vi "Get Settings File Name.vi"(7 "Source Path":path, 8 "error in (no error)":errorcluster) -> (0 "error out":errorcluster, 1 "Cancelled":bool, 2 "Sink File":string, 3 "Sink Folder":path)   [LabVIEW 2019, in "Test Executive Explorer.lvclass"]
uses:
  <vilib>/gpm_packages/@cs/Test-executive-builder/Example/Application/Test Executive Explorer/Test Executive Explorer/Test Executive Explorer.lvclass
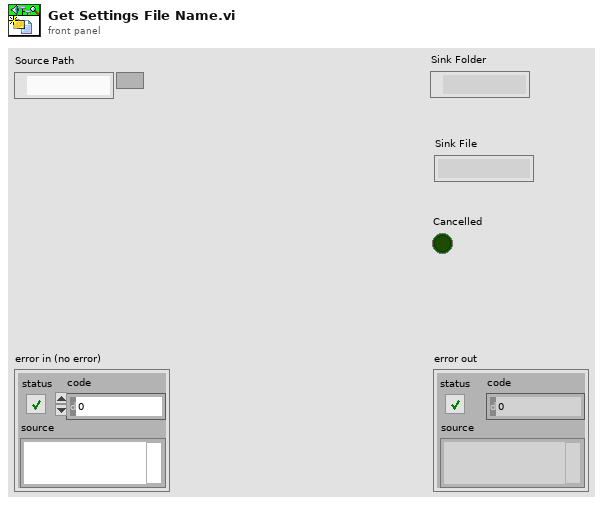
[diagram p1: front panel]
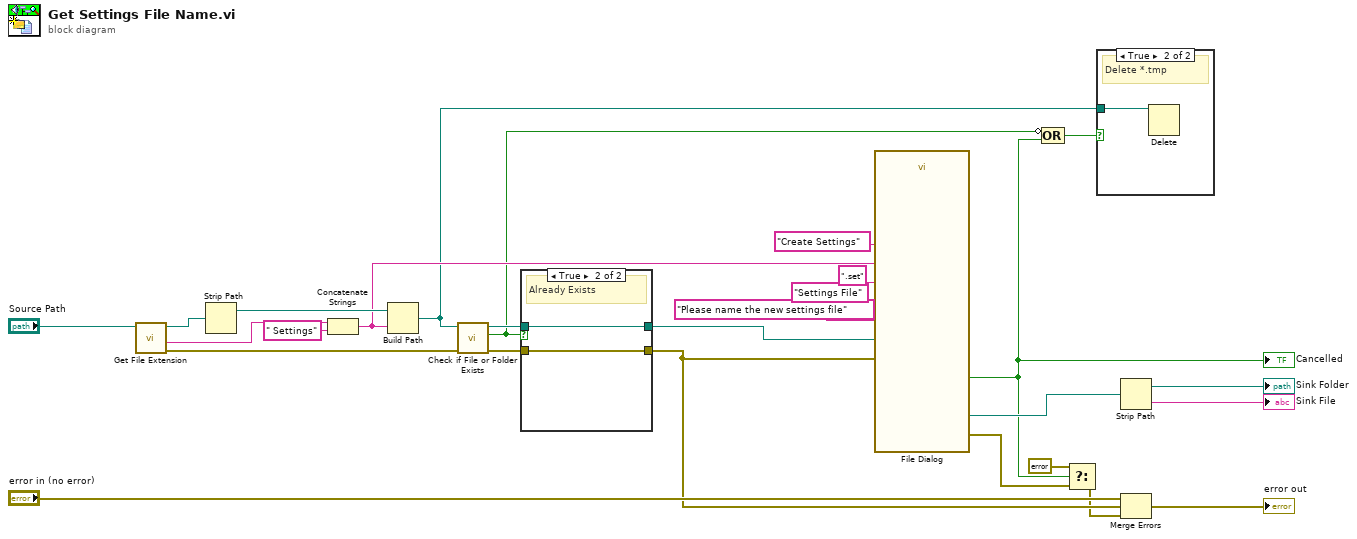
[diagram p0: block diagram]
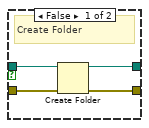
[diagram p3: hidden frame]
diagram:
  n1 = call <vilib>:"Get File Extension.vi"("file"="Source Path") -> ("error out"=w22:errorcluster, "filename without extension"=w25:string, "dup file"=w26:path)  [unwired: 6 in, 2 out]
  n2 = Strip Path(path=w26) -> (stripped path=w23:path)  [unwired: 1 out]
  n3 = Concatenate Strings(w25, " Settings" ("string")) -> (w12:string)
  n4 = Build Path(base path=w23, name or relative path=w12) -> (appended path=w1:path)
  n5 = call <vilib>:"Check if File or Folder Exists.vi"("error in (no error)"=w22, "path"=w1) -> ("error out"=w20:errorcluster, "file or folder exists?"=w3:bool, "dup path"=w21:path)  [unwired: 7 in]
  n6 = case shown="True" w3 {
    tunnel: w21 -> [w31 w33]
    tunnel: w20 -> [w30 w32]
    tunnel: [w29 w33] -> w19
    tunnel: [w28 w32] -> w14
    frame False {
      # "Create Folder"
      n7 = Create Folder(path (use dialog)=w31, error in=w30) -> (created path=w29:path, error out=w28:errorcluster)  [unwired: 1 in, 1 out]
    }
    frame True {
      # "Already Exists"
    }
  }
  n8 = call "File Dialog"("start path"=w19, "prompt"="Please name the new settings file", "button label"="Create Settings", "default name"=w12, "error in"=w14, "pattern (all files)"=".set", "pattern label"="Settings File") -> ("selected path"=w18:path, "cancelled"=w4:bool, "error out"=w8:errorcluster)  [unwired: 5 in, 1 out]
  "Cancelled" <- w4
  n9 = Compound Arithmetic op=OR(invert w3, w4) -> (w2:bool)
  n10 = Select(t=errorcluster {"status"=FALSE, "code"=0, "source"=""}, s=w4, f=w8) -> (s? t:f=w5:errorcluster)
  n11 = case shown="True" w2 {
    tunnel: w1 -> [_ w34]
    frame False {
    }
    frame True {
      # "Delete *.tmp"
      n12 = Delete(path (use dialog)=w34) -> ()  [unwired: 4 in, 3 out]
    }
  }
  n13 = Strip Path(path=w18) -> (stripped path=→"Sink Folder":path, name=→"Sink File":string)
  n14 = Merge Errors("error in (no error)", w14, w5) -> (→"error out":errorcluster)
